vi "Iterate.vi"(10 "Iterate":i32, 11 "Iterate in":refnum<class "Iterate.lvclass">) -> (3 "Iterate out":refnum<class "Iterate.lvclass">)   [LabVIEW 2021, in "Hello World Event.lvlib" / "Iterate Msg Strategy.lvlib" / "Iterate.lvclass"]
uses:
  Iterate.lvclass
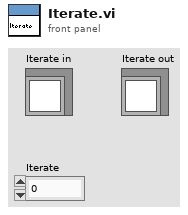
[diagram p1: front panel]
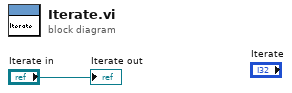
[diagram p0: block diagram]
diagram:
  "Iterate out" <- "Iterate in"
